vi "Intake Set.vi"(1 "Intake Info In":T2) -> (0 "Intake Info Out":T2)   [LabVIEW 2013]
uses:
  <vilib>/Rock Robotics/WPI/Solenoid/WPI_SolenoidValue.ctl
  <vilib>/Rock Robotics/WPI/Solenoid/WPI_SolenoidSetEnum.vi
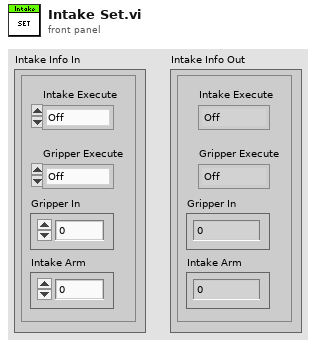
[diagram p1: front panel]
types:
  T1 = typedef "WPI_SolenoidValue.ctl" = enum16{"Off", "On", "Forward", "Reverse"}
  T2 = cluster{"Intake Execute":T1, "Gripper Execute":T1, "Gripper In":dbl, "Intake Arm":dbl}
  T3 = typedef "WPI_SolenoidDevRef.ctl" = cluster{"DevStatus":errorcluster, "Solenoid Module":T4, "Forward Solenoid Channel":T5, "Reverse Solenoid Channel":T5}
  T4 = typedef "FPGA_TypedefSolenoidModule.ctl" = enum16{"Solenoid Module 1", "Solenoid Module 2"}
  T5 = typedef "WPI_SolenoidChannel.ctl" = enum8{"Solenoid 1", "Solenoid 2", "Solenoid 3", "Solenoid 4", "Solenoid 5", "Solenoid 6", "Solenoid 7", "Solenoid 8", "Invalid"}
  T6 = typedef "WPI_RelayDevRef.ctl" = cluster{"DevStatus":errorcluster, "Relay Channel":T7, "Digital Module":T8, "Relay Direction":T9}
  T7 = typedef "FPGA_DIORelayChannel.ctl" = enum8{"Relay 1", "Relay 2", "Relay 3", "Relay 4", "Relay 5", "Relay 6", "Relay 7", "Relay 8", "Invalid"}
  T8 = typedef "FPGA_TypedefDigitalModule.ctl" = enum16{"Digital Module 1", "Digital Module 2"}
  T9 = typedef "WPI_RelayDirection.ctl" = enum16{"Both directions", "Forward only", "Reverse only"}
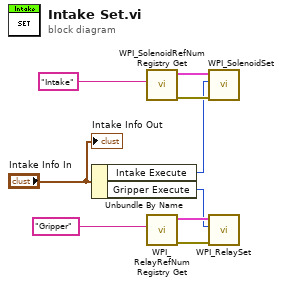
[diagram p0: block diagram]
diagram:
  n1 = Unbundle By Name("Intake Info In") -> ("Intake Execute"=w2:T1, "Gripper Execute"=w6:T1)
  n2 = call <vilib>:"WPI_SolenoidRefNum Registry Get.vi"("refnum name"="Intake") -> ("error out"=w4:errorcluster, "SolenoidDevRef"=w3:T3)  [unwired: 9 in]
  n3 = call <vilib>:"WPI_RelayRefNum Registry Get.vi"("refnum name"="Gripper") -> ("error out"=w7:errorcluster, "RelayDevRef"=w8:T6)  [unwired: 9 in]
  n4 = call-poly <vilib>:"WPI_SolenoidSet.vi"("error in (no error)"=w4, "Value"=w2, "SolenoidDevRef"=w3) -> ()  [unwired: 7 in, 2 out]
  n5 = call <vilib>:"WPI_RelaySet.vi"("error in (no error)"=w7, "RelayValue"=w6, "RelayDevRef"=w8) -> ()  [unwired: 7 in, 2 out]
  "Intake Info Out" <- "Intake Info In"
